vi "Write Acquisition Complete.vi"(8 "error in (no error)":errorcluster, 10 "Acquisition Complete":bool, 11 "Scope Instrument in":refnum<class "Scope Instrument.lvclass">) -> (0 "error out":errorcluster, 3 "Scope Instrument out":refnum<class "Scope Instrument.lvclass">)   [LabVIEW 2025, in "Scope.lvlib" / "Scope Instrument.lvclass"]
uses:
  Scope Instrument.lvclass
  Scope Instrument.lvclass/Scope Instrument.ctl
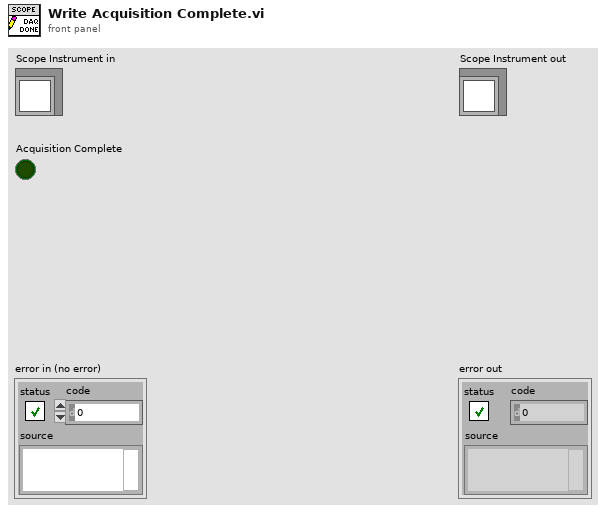
[diagram p1: front panel]
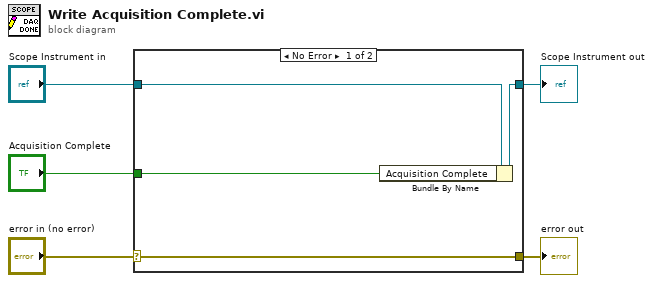
[diagram p0: block diagram]
diagram:
  n1 = case shown="No Error" "error in (no error)" {
    selector: "error in (no error)" -> [w9 w10]
    tunnel: [w9 w10] -> w4
    tunnel: [w7 w11] -> w2
    tunnel: "Scope Instrument in" -> [w8 w11]
    tunnel: "Acquisition Complete" -> [w6 _]
    frame No Error {
      n2 = Bundle By Name(cluster=w8, "Acquisition Complete"=w6) -> (w7:refnum<class "Scope Instrument.lvclass">)
    }
    frame Error {
    }
  }
  "error out" <- w4
  "Scope Instrument out" <- w2
